vi "Select Sheet.vi"(7 "Sheet (0)":i32, 8 "error in (no error)":errorcluster, 11 "IWorkbook Reference":refnum<k24>) -> (0 "error out":errorcluster, 2 "Sheet Reference":refnum<k24>, 3 "IWorkbook Reference":refnum<k24>)   [LabVIEW 2014]
uses:
  C:/Users/LENOVO/Desktop/CodeSpace GUI/LVExcel/Resources/net40/NPOI.dll
  Resources/net40/NPOI.dll
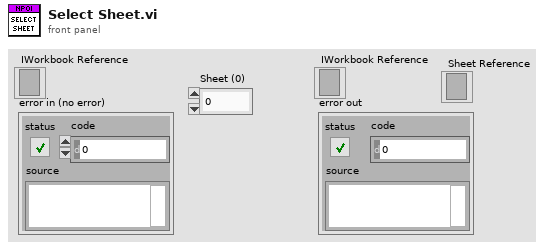
[diagram p1: front panel]
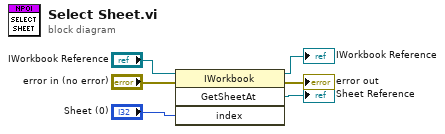
[diagram p0: block diagram]
diagram:
  n1 = invoke class="IWorkbook" method="GetSheetAt"(reference="IWorkbook Reference", error in="error in (no error)", "index"="Sheet (0)") -> (reference out=→"IWorkbook Reference":refnum<k24>, error out=→"error out":errorcluster, "GetSheetAt"=→"Sheet Reference":refnum<k24>)  [unwired: 1 in, 1 out]
